vi "Initialize.vi"(8 "error in (no error)":errorcluster, 9 "Reset (T: Reset)":bool=TRUE, 10 "ID Query (T: Check)":bool=TRUE, 11 "VISA resource name":refnum<visa-resource-name>) -> (0 "error out":errorcluster, 3 "VISA resource name out":refnum<visa-resource-name>)   [LabVIEW 2016, in "Agilent 428X Series.lvlib"]
doc: "This VI passes the addressing information in the instrument decriptor to the Instr Open VI and returns the instrument ID. You can optionally reset the instrument by setting the front panel reset control. You must run this VI before using any of the instrument driver VIs for this instrument."
uses:
  <instrlib>/Agilent 428X Series/Agilent 428X Series.lvlib
panel:
  # "© Copyright 2005 National Instruments Corporation.  All Rights Reserved."
  # "Check\nDon't Check"
  # "Reset\nDon't Reset"
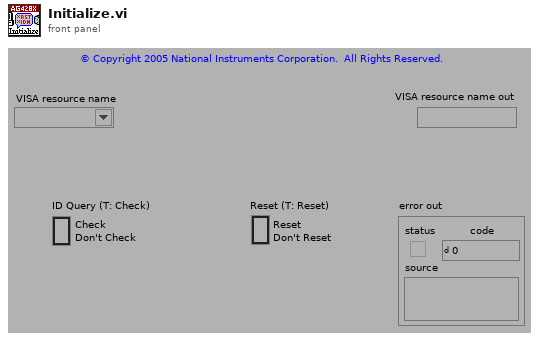
[diagram p1: front panel]
types:
  T1 = cluster{"status":bool, "code":i32, "VI name":string}
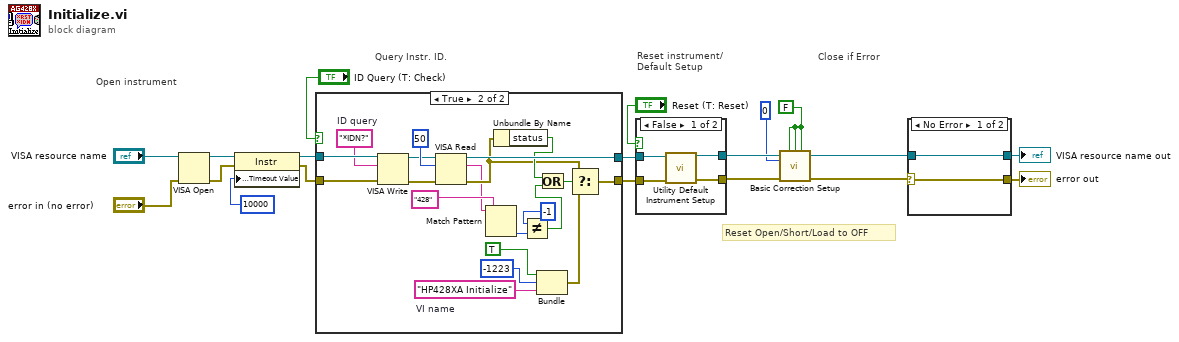
[diagram p0: block diagram]
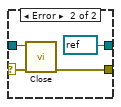
[diagram p2: hidden frame]
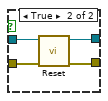
[diagram p3: hidden frame]
diagram:
  w4 = FALSE
  # "Reset Open/Short/Load to OFF"
  # "Close if Error"
  # "Query Instr. ID."
  # "Reset instrument/\nDefault Setup"
  # "Open instrument"
  n1 = VISA Open(error in (no error)="error in (no error)", VISA resource name="VISA resource name") -> (VISA resource name=w9:refnum<visa-resource-name>, error out=w11:errorcluster)  [unwired: 3 in]
  n2 = property class="Instr"(reference=w9, error in=w11, "General Settings:Timeout Value"=u32 10000 ("Tmo Value")) -> (reference out=w8:refnum<visa-resource-name>, error out=w10:errorcluster)
  n3 = case shown="True" "ID Query (T: Check)" {
    tunnel: [w20 w41] -> w18
    tunnel: [w21 w38] -> w19
    tunnel: w8 -> [w21 w39]
    tunnel: w10 -> [w20 w40]
    frame False {
    }
    frame True {
      w34 = "*IDN?"  # ID query
      w22 = "HP428XA Initialize"  # VI name
      n4 = VISA Write(VISA resource name=w39, write buffer=w34, error in (no error)=w40) -> (VISA resource name out=w25:refnum<visa-resource-name>, error out=w27:errorcluster)  [unwired: 1 out]
      n5 = VISA Read(VISA resource name=w25, byte count=u32 50, error in (no error)=w27) -> (VISA resource name out=w38:refnum<visa-resource-name>, read buffer=w24:string, error out=w26:errorcluster)  [unwired: 1 out]
      n6 = Match Pattern(string=w24, regular expression="428") -> (offset past match=w32:i32)  [unwired: 1 in, 3 out]
      n7 = Unbundle By Name(w26) -> ("status"=w29:bool)
      n8 = Not Equal?(x=-1, y=w32) -> (x != y?=w23:bool)
      n9 = Bundle(TRUE, -1223, "VI name"=w22) -> (w35:cluster{bool, i32, "VI name":string})  [unwired: 1 in]
      n10 = Or(x=w29, y=w23) -> (x .or. y?=w28:bool)
      n11 = Select(t=w26, s=w28, f=w35) -> (s? t:f=w41:T1)
    }
  }
  n12 = case shown="False" "Reset (T: Reset)" {
    tunnel: w18 -> [w44 w48]
    tunnel: [w43 w46] -> w6
    tunnel: w19 -> [w45 w49]
    tunnel: [w42 w47] -> w7
    frame False {
      n13 = call <instrlib>:"Utility Default Instrument Setup.vi"("error in (no error)"=w44, "VISA resource name"=w45) -> ("error out"=w43:errorcluster, "VISA resource name out"=w42:refnum<visa-resource-name>)  [unwired: 8 in]
    }
    frame True {
      n14 = call <instrlib>:"Reset.vi"("error in (no error)"=w48, "VISA resource name"=w49) -> ("error out"=w46:errorcluster, "VISA resource name out"=w47:refnum<visa-resource-name>)  [unwired: 8 in]
    }
  }
  n15 = call <instrlib>:"Basic Correction Setup.vi"("VISA resource name"=w7, "Load Corr  (F: Off)"=w4, "Short Corr (T: On)"=w4, "Open Corr  (F: Off)"=w4, "Cable Length (0: 4 m)"=u32 0 ("Cable Length (0: 0 m)"), "error in (no error)"=w6) -> ("VISA resource name out"=w3:refnum<visa-resource-name>, "error out"=w1:errorcluster)  [unwired: 7 in, 1 out]
  n16 = case shown="No Error" w1 {
    selector: w1 -> [w50 w52]
    tunnel: w3 -> [w51 w55]
    tunnel: [w51 refnum<visa-resource-name> refnum ("dup VISA session")] -> w14
    tunnel: [w50 w54] -> w13
    frame No Error {
    }
    frame Error {
      n17 = call <instrlib>:"Close.vi"("error in (no error)"=w52, "VISA resource name"=w55) -> ("error out"=w54:errorcluster)  [unwired: 9 in]
    }
  }
  "VISA resource name out" <- w14
  "error out" <- w13
